vi "estimate_stopp_time.vi"(9 "Aktueller Messschritt":i32, 10 "# Messschritte":i32, 11 "Startzeit":timestamp) -> (3 "Stopp Zeit":string)   [LabVIEW 2009]
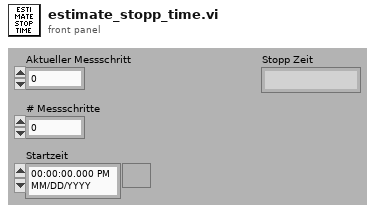
[diagram p1: front panel]
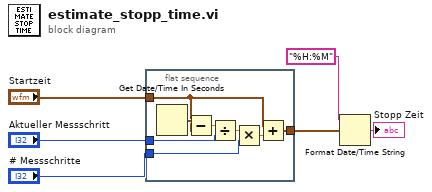
[diagram p0: block diagram]
diagram:
  n1 = flat-sequence {
    tunnel: "Startzeit" -> [w7]
    tunnel: "Aktueller Messschritt" -> [w13]
    tunnel: "# Messschritte" -> [w11]
    tunnel: [w8] -> w2
    frame #0 {
      n2 = Get Date/Time In Seconds() -> (seconds since 1Jan1904=w10:timestamp)
      n3 = Subtract(x=w10, y=w7) -> (x-y=w14:dbl)
      n4 = Divide(x=w14, y=w13) -> (x/y=w12:dbl)
      n5 = Multiply(x=w12, y=w11) -> (x*y=w9:dbl)
      n6 = Add(x=w7, y=w9) -> (x+y=w8:timestamp)
    }
  }
  n7 = Format Date/Time String(time format string (%c)="%H:%M" ("Zeitformatierungs-String (%c)"), seconds (now)=w2) -> (date/time string=→"Stopp Zeit":string)  [unwired: 1 in]
